vi "convert WF to image.vi"(5 "analysis result":T1, 6 "Array Wavefront in":sgl[](array[numeric]), 7 "VISA Refnum in":refnum<visa-resource-name>, 8 "error in (no error)":errorcluster, 9 "Value 2":dbl, 10 "Value":dbl, 11 "Refnum in":T2) -> (0 "error out":errorcluster, 1 "Array Wavefront out":sgl[][](array[numeric]), 2 "instrument handle out":refnum<visa-resource-name>, 3 "Refnum out":T2, 4 "output cluster":T1)   [LabVIEW 2020, in "ThorlabsWFS.lvclass"]
uses:
  ThorlabsWFS.lvclass
  <vilib>/vision/Image Controls.llb/IMAQ Image.ctl
  analysis result.ctl
  <vilib>/vision/NI_Vision_Development_Module.lvlib
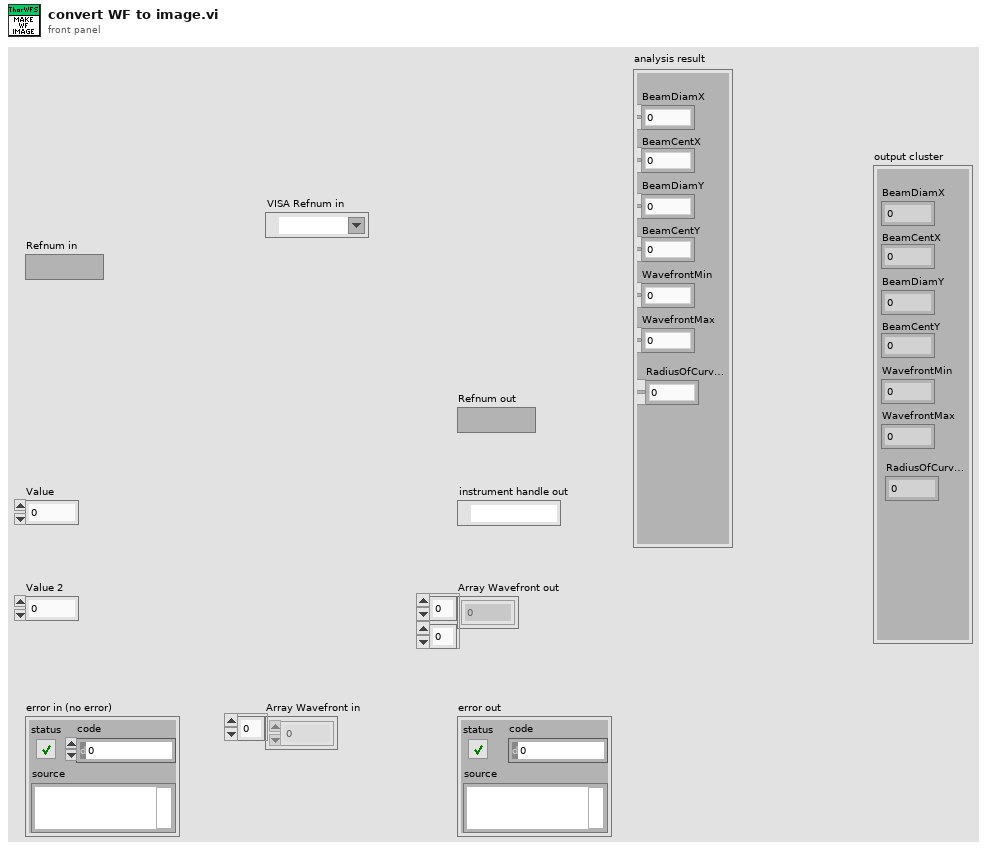
[diagram p1: front panel]
types:
  T1 = typedef "ThorlabsWFS.lvclass/analysis result.ctl" = cluster{"BeamDiamX":dbl, "BeamCentX":dbl, "BeamDiamY":dbl, "BeamCentY":dbl, "WavefrontMin":dbl, "WavefrontMax":dbl, "RadiusOfCurvature":dbl}
  T2 = typedef "IMAQ Image.ctl" = refnum<image>
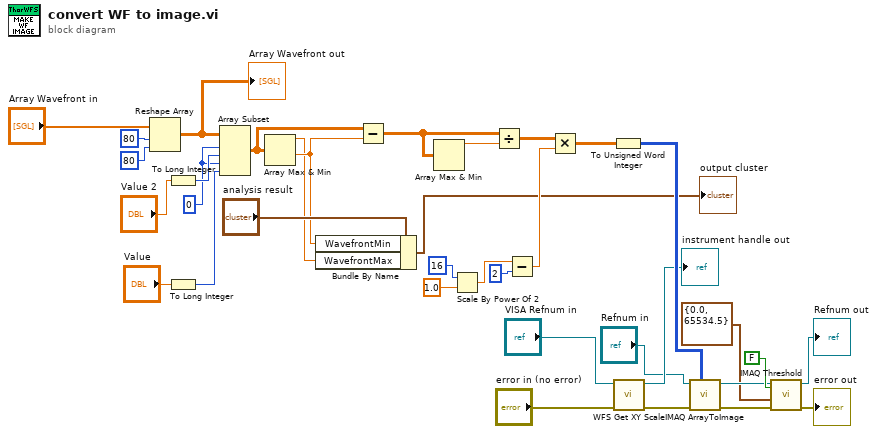
[diagram p0: block diagram]
diagram:
  w13 = 0 ("index")
  n1 = Reshape Array("Array Wavefront in", 80 ("dimension size"), 80 ("dimension size")) -> (w16:sgl[][])
  "Array Wavefront out" <- w16
  n2 = To Long Integer(number="Value 2") -> (32bit integer=w14:i32)
  n3 = To Long Integer(number="Value") -> (32bit integer=w15:i32)
  n4 = Array Subset(array=w16, index (row)=w13, length (row)=w14, index (col)=w13, length (col)=w15) -> (w6:sgl[][])
  n5 = Array Max & Min(array=w6) -> (max value=w3:sgl, min value=w4:sgl)  [unwired: 2 out]
  n6 = Bundle By Name(cluster="analysis result", "WavefrontMin"=w4, "WavefrontMax"=w3) -> (→"output cluster":T1)
  n7 = Subtract(x=w6, y=w4) -> (x-y=w27:sgl[][])
  n8 = Array Max & Min(array=w27) -> (max value=w26:sgl)  [unwired: 3 out]
  n9 = Scale By Power Of 2(n=i16 16, x=1.0) -> (x*2^n=w32:dbl)
  n10 = Divide(x=w27, y=w26) -> (x/y=w28:sgl[][])
  n11 = Subtract(x=w32, y=2) -> (x-y=w33:dbl)
  n12 = Multiply(x=w28, y=w33) -> (x*y=w34:dbl[][])
  n13 = To Unsigned Word Integer(number=w34) -> (unsigned 16bit integer=w35:u16[][])
  n14 = call "WFS Get XY Scale.vi"("error in (no error)"="error in (no error)", "instrument handle"="VISA Refnum in") -> ("error out"=w21:errorcluster, "instrument handle out"=→"instrument handle out":refnum<visa-resource-name>)  [unwired: 6 in, 2 out]
  n15 = call "IMAQ ArrayToImage"("Image Pixels (U16)"=w35, "error in (no error)"=w21, "Image"="Refnum in") -> ("error out"=w22:errorcluster, "Image Out"=w24:T2)  [unwired: 7 in]
  n16 = call "IMAQ Threshold"("Keep/Replace Value (Replace)"=FALSE, "error in (no error)"=w22, "Range"=cluster{"Lower value":sgl, "Upper value":sgl} {"Lower value"=0.0, "Upper value"=65534.5}, "Image Src"=w24) -> ("error out"=→"error out":errorcluster, "Image Dst Out"=→"Refnum out":T2)  [unwired: 6 in]
